vi "INIT_GenerateConfigurationFolderPath.vi"(7 "Top VI Path":path) -> (4 "Configuration Folder Path (String Format)":string, 15 "Configuration Folder Path":path)   [LabVIEW 2024]
doc: "Formats the path to the Configuration Folder depends from the type and location of the top level (RCPVMS) VI."
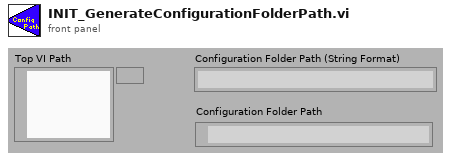
[diagram p1: front panel]
types:
  T1 = enum32{"invalid app kind", "Development System", "Run Time System", "Student Edition", "Embedded LabVIEW", "Evaluation", "Custom"}
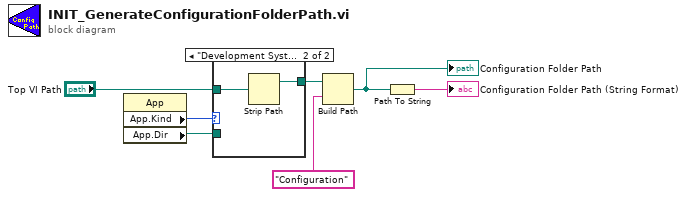
[diagram p0: block diagram]
diagram:
  n1 = property on="Property Node" class="App"() -> ("App.Kind"=w2:T1, "App.Dir"=w1:path)  [unwired: 2 in, 2 out]
  n2 = case shown="\"Development System\", \"Evaluation\"" w2 {
    tunnel: "Top VI Path" -> [_ w9]
    tunnel: w1 -> [w8 _]
    tunnel: [w8 w10] -> w6
    frame "Run Time System", Default {
    }
    frame "Development System", "Evaluation" {
      n3 = Strip Path(path=w9) -> (stripped path=w10:path)  [unwired: 1 out]
    }
  }
  n4 = Build Path(base path=w6, name or relative path="Configuration" ("string")) -> (appended path=w3:path)
  "Configuration Folder Path" <- w3
  n5 = Path To String(path=w3) -> (string=→"Configuration Folder Path (String Format)":string)
